vi "Best y for any element.vi"(7 "Enemys(T)\nAllys(F)":bool=TRUE, 9 "Maior intervalo(T)\nMaior angulo(F)":bool, 10 "IA State":T2={"our_robots"=[], "enemy_robots"=[], "balls"=[], "geometry"={"line_width"=0, "field_length"=0, "field_width"=0, "boundary_width"=0, "referee_width"=0, "goal_width"=0, "goal_depth"=0, "goal_wall_width"=0, "center_circle_radius"=0, "defense_radius"=0, "defense_stretch"=0, "free_kick_from_defense_dist"=0, "penalty_spot_from_field_line_dist"=0, "penalty_line_from_spot_dist"=0}, "IA Judge"={"stage"="", "command"="", "our_goalie_id"=0.0, "enemy_goalie_id"=0.0, "command enum"=enum."Halt", "Time"=enum."Azul"}, "Received Timestamp"=timestamp(0 s since 1904-01-01), "Events"={"Touch"=FALSE, "Ball out"=FALSE, "id touch"=0.0, "Ball out of \nVision"=FALSE, "Ball inside \nGoalie area"=FALSE, "Robot not responding"=FALSE, "Robots responding status"=[1.0, 1.0, 1.0, 1.0, 1.0, 1.0], "Enemy Ball \nPossession"=FALSE, "Pass State"=FALSE, "id end of pass"=0.0, "Kick"=FALSE, "Id ini Possession"=0.0, "Ball Possesion"=FALSE, "Id Possesion"=0.0, "Direct Kick"=FALSE, "2nd Strk Ativo"=FALSE}}, 11 "Element Position":dbl[](array[numeric])) -> (1 "Goal Gap Normalizado(%do gol aberta)":dbl, 2 "Best y(for kick target)":dbl, 3 "Goal Gap":dbl, 4 "Eclipse":bool, 5 "Gap Coord":dbl[](array[numeric]))   [LabVIEW 2017]
uses:
  Core/AI Input.ctl
  Core/AI Robot.ctl
  Intel/Functions Enum.ctl
  Intel/AttackerStates.ctl
  Path Planning/RRT/PathDests.ctl
  Path Planning/RRT/PathDest.ctl
  Core/AI Ball.ctl
  Core/Field Size.ctl
  Core/AI Judge.ctl
  Intel/Command Enum.ctl
  Events/Events.ctl
  segment.ctl
  <vilib>/Analysis/baseanly.llb/Real Dot Product.vi
  <vilib>/Analysis/NI_AALBase.lvlib
panel:
  out "Vetor de gaps \ncorreto":T1[](array[typedef])
  out "Vetor de gaps":T1[](array[typedef])
  in  "eclipse angle eps":dbl=0.035 format="%#_13g"
  out "pilha output (merged)":T1[](array[typedef])
  out "Vetor de segmentos ordenado":T1[](array[typedef])
  out "Vetor de segmentos (sombras)":T1[](array[typedef])
  # "Default FALSE"
  # "Quem será considerado obstaculo"
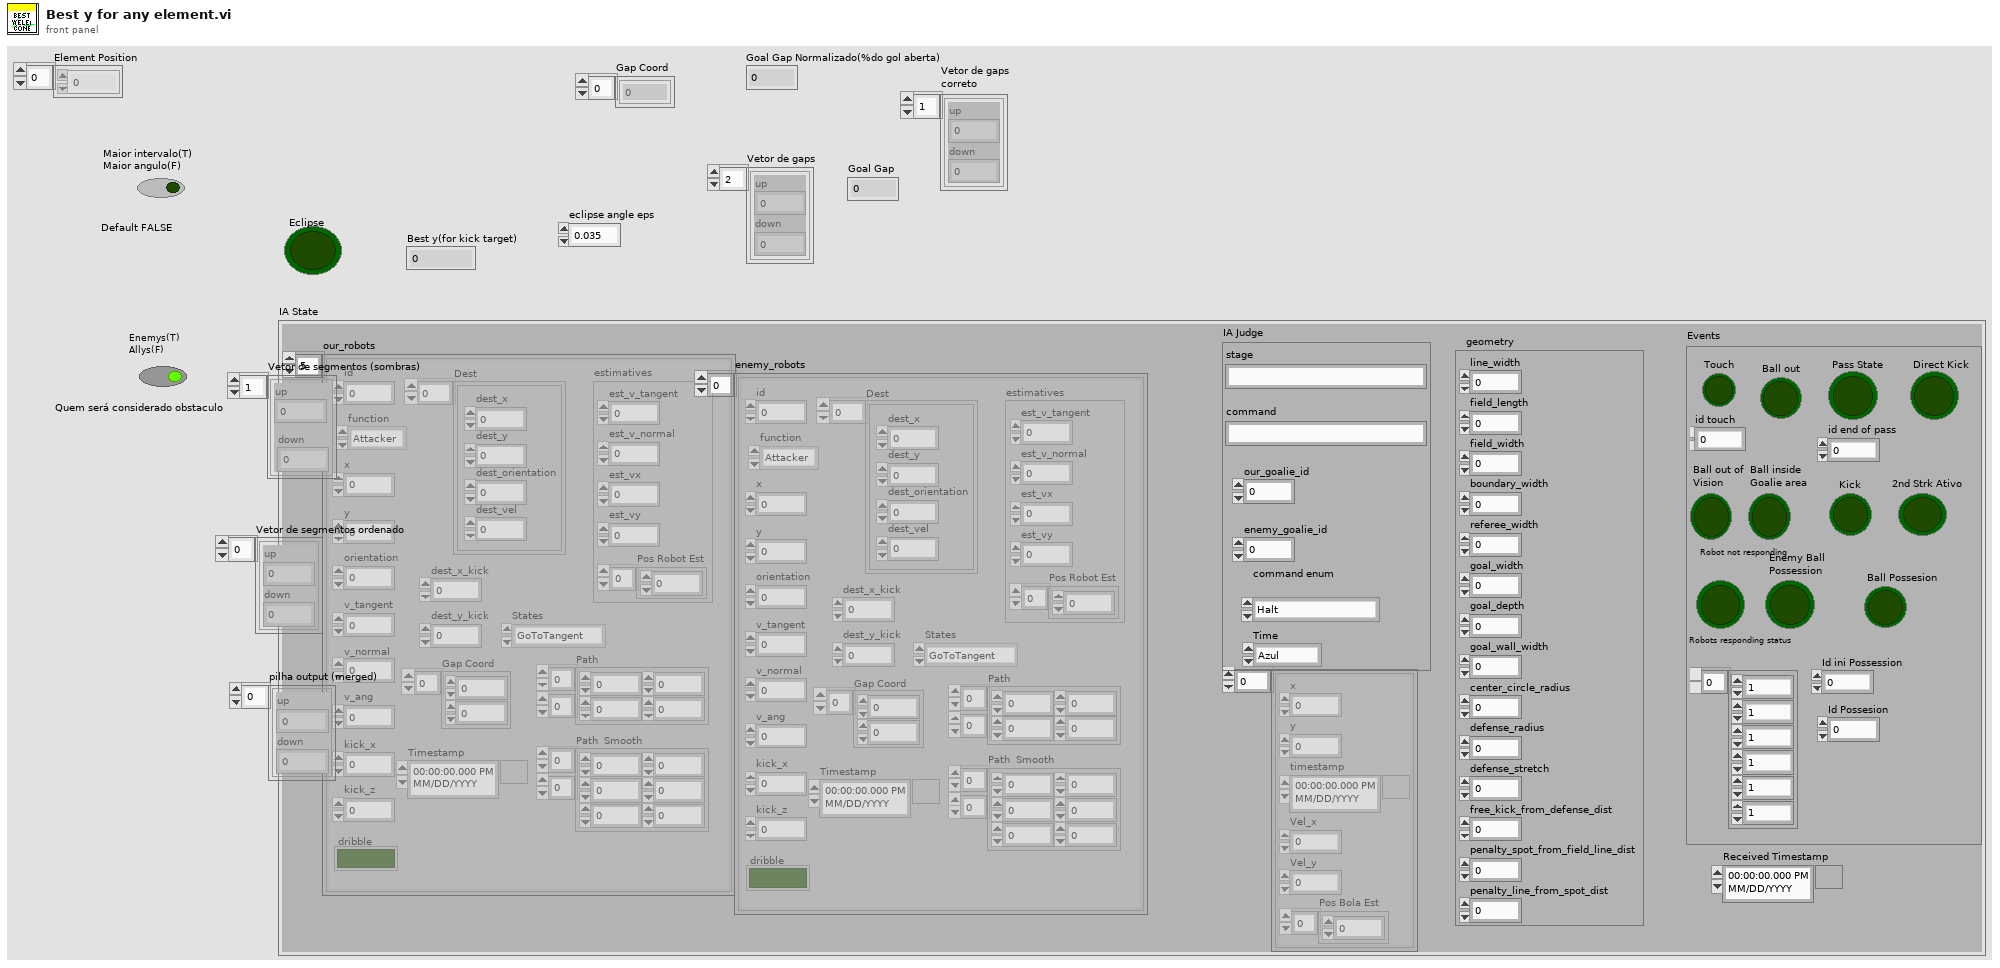
[diagram p1: front panel]
types:
  T1 = typedef "segment.ctl" = cluster{"up":dbl, "down":dbl}
  T2 = typedef "AI Input.ctl" = cluster{"our_robots":T3[], "enemy_robots":T3[], "balls":T8[], "geometry":T9, "IA Judge":T10, "Received Timestamp":timestamp, "Events":T12}
  T3 = typedef "AI Robot.ctl" = cluster{"id":u32, "function":T4, "x":dbl, "y":dbl, "orientation":dbl, "v_tangent":dbl, "v_normal":dbl, "v_ang":dbl, "kick_x":dbl, "kick_z":dbl, "dribble":bool, "Timestamp":timestamp, "estimatives":cluster{"est_v_tangent":dbl, "est_v_normal":dbl, "est_vx":dbl, "est_vy":dbl, "Pos Robot Est":dbl[]}, "dest_x_kick":dbl, "dest_y_kick":dbl, "Gap Coord":dbl[], "States":T5, "Path ":dbl[][], "Path  Smooth":dbl[][], "Dest":T6}
  T4 = typedef "Functions Enum.ctl" = enum16{"2nd Striker", "Attacker", "Goalie", "Defender", "Striker", "Goto 0", "Dummy", "Kicker", "ZigZag 0", "ZigZag 1", "ZigZag 2", "ZigZag 3", "ZigZag 4", "ZigZag 5", "ZigZag 6", "ZigZag 7", "ZigZag 8", ""}
  T5 = typedef "AttackerStates.ctl" = enum16{"Pass", "GoToTangent", "BallGetting", "GoToKick", ""}
  T6 = typedef "PathDests.ctl" = T7[]
  T7 = typedef "PathDest.ctl" = cluster{"dest_x":dbl, "dest_y":dbl, "dest_orientation":dbl, "dest_vel":dbl}
  T8 = typedef "AI Ball.ctl" = cluster{"x":dbl, "y":dbl, "timestamp":timestamp, "Vel_x":dbl, "Vel_y":dbl, "Pos Bola Est":dbl[]}
  T9 = typedef "Field Size.ctl" = cluster{"line_width":u32, "field_length":u32, "field_width":u32, "boundary_width":u32, "referee_width":u32, "goal_width":u32, "goal_depth":u32, "goal_wall_width":u32, "center_circle_radius":u32, "defense_radius":u32, "defense_stretch":u32, "free_kick_from_defense_dist":u32, "penalty_spot_from_field_line_dist":u32, "penalty_line_from_spot_dist":u32}
  T10 = typedef "AI Judge.ctl" = cluster{"stage":string, "command":string, "our_goalie_id":dbl, "enemy_goalie_id":dbl, "command enum":T11, "Time":enum16{"Azul", "Amarelo"}}
  T11 = typedef "Command Enum.ctl" = enum16{"Halt", "Stop", "Force Start", "PKA Normal Start", "Prepare Kickoff Ally", "PKE Normal Start", "Prepare Kickoff Enemy", "Prepare Penalty Ally", "PPA Normal Start", "Prepare Penalty Enemy", "PPE Normal Start", "Direct Free Enemy", "Direct Free Ally", "Indirect Free Enemy", "Indirect Free Ally", "Timeout Enemy", "Timeout Ally", "Goal Enemy", "Goal Ally", "Ball Placement Enemy", "Ball Placement Ally", "Normal Half Time", "Extra Time Break", "Extra Half Time", "None", "Post Game"}
  T12 = typedef "Events.ctl" = cluster{"Touch":bool, "Ball out":bool, "id touch":dbl, "Ball out of \nVision":bool, "Ball inside \nGoalie area":bool, "Robot not responding":bool, "Robots responding status":dbl[], "Enemy Ball \nPossession":bool, "Pass State":bool, "id end of pass":dbl, "Kick":bool, "Id ini Possession":dbl, "Ball Possesion":bool, "Id Possesion":dbl, "Direct Kick":bool, "2nd Strk Ativo":bool}
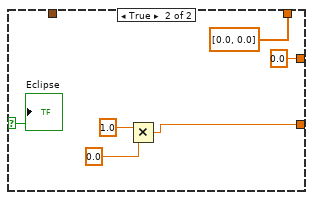
[diagram p4: hidden frame]
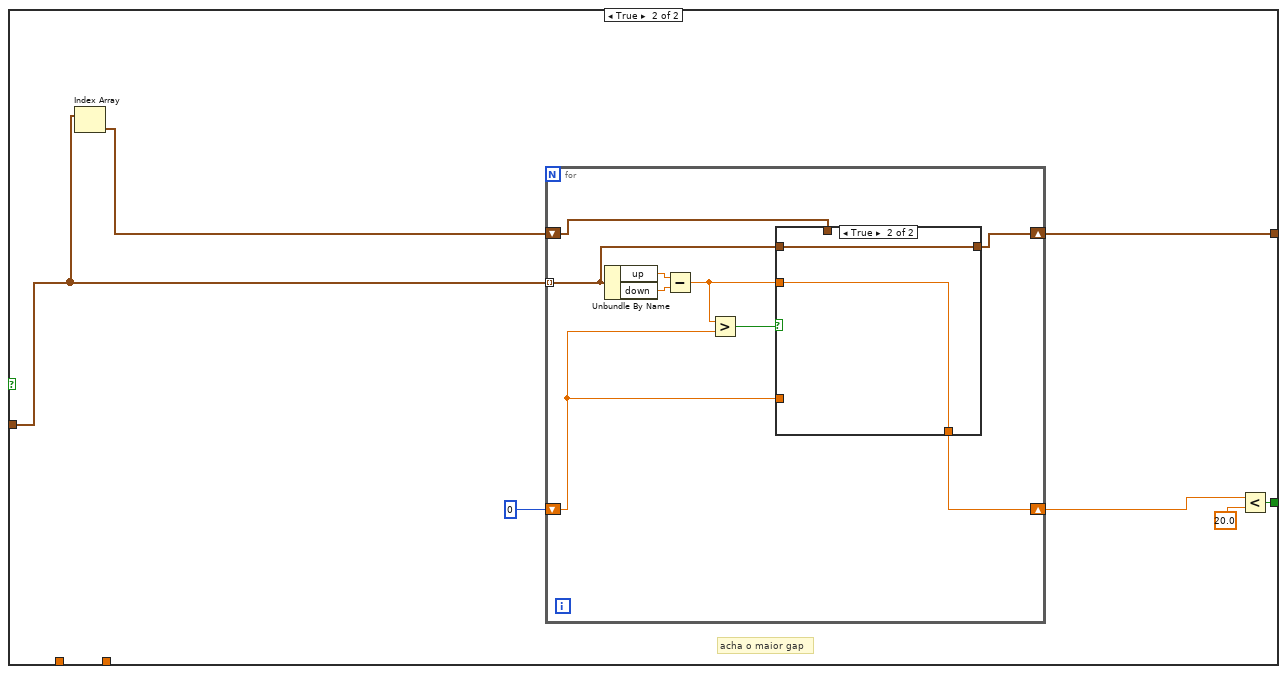
[diagram p6: hidden frame]
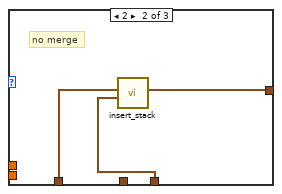
[diagram p8: hidden frame]
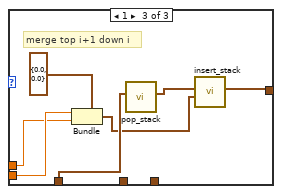
[diagram p9: hidden frame]
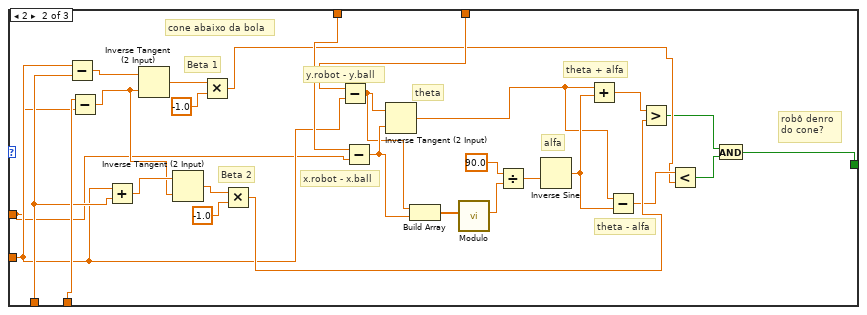
[diagram p11: hidden frame]
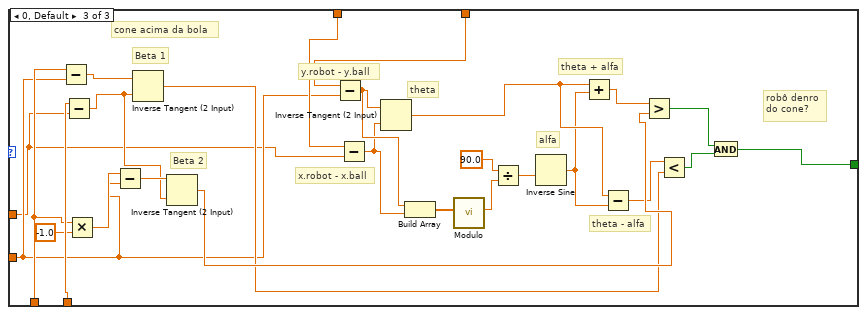
[diagram p12: hidden frame]
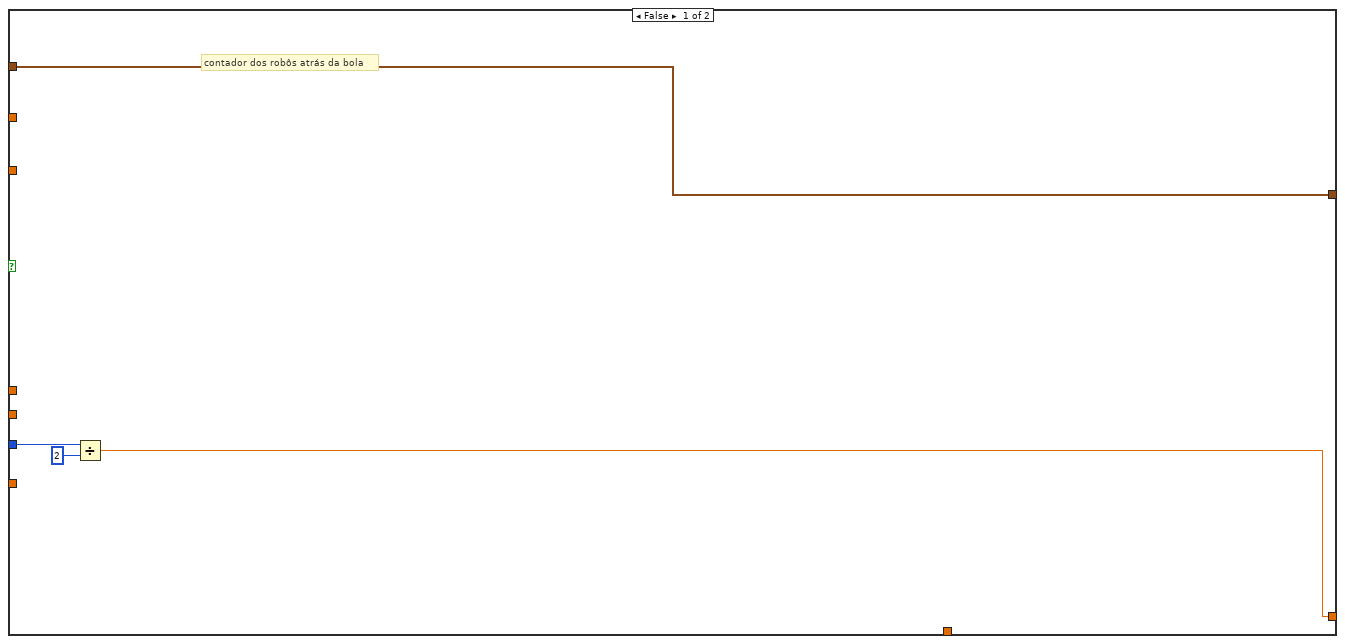
[diagram p13: hidden frame]
diagram:
  # "default T"
  # "Default FALSE"
  # "goal_width/2"
  # "field_length/2"
  # "balls"
  # "vetor de gaps"
  # "upper"
  n1 = Unbundle By Name("IA State") -> ("enemy_robots"=w21:T3[], "our_robots"=w20:T3[])
  n2 = Unbundle By Name("IA State") -> ("geometry.field_length"=w39:u32, "geometry.goal_width"=w2:u32)
  n3 = Select(t=w21, s="Enemys(T)\nAllys(F)", f=w20) -> (s? t:f=w19:T3[])
  n4 = Divide(x=w2, y=u32 2 ("x")) -> (x/y=w10:dbl)
  n5 = To Double Precision Float(number=w2) -> (double precision float=w1:dbl)
  n6 = for {
    shift-right: [w74] -> w24
    shift-left: T1[] [] -> [w73]
    tunnel: w39 -> [w51]
    tunnel: w10 -> [w53]
    tunnel: w10 -> [w71]
    shift-right: [w70] -> w22
    shift-left: _ -> [_]
    tunnel: w19 -> [w69] mode=indexing
    tunnel: "Enemys(T)\nAllys(F)" -> [w67]
    tunnel: "Element Position" -> [w43]
    # "y element"
    # "x element"
    # "y.robot"
    # "x.robot"
    # "field_length/2"
    # "goal_width/2"
    # "y element"
    # "x element"
    n7 = Index Array(array=w43) -> (element #1=w42:dbl, element #2=w41:dbl)  [unwired: 2 in]
    n8 = Unbundle By Name(w69) -> ("x"=w49:dbl, "y"=w48:dbl)
    n9 = Multiply(x=w49, y=-1.0) -> (x*y=w66:dbl)
    n10 = Absolute Value(x=w42) -> (abs(x)=w65:dbl)
    n11 = Absolute Value(x=w49) -> (abs(x)=w72:dbl)
    n12 = Select(t=w49, s=w67, f=w66) -> (s? t:f=w46:dbl)
    n13 = Greater?(x=w72, y=w65) -> (0:w44:bool)
    n14 = Multiply(x=w53, y=-1.0) -> (x*y=w57:dbl)
    n15 = Greater?(x=w41, y=w53) -> (0:w56:bool)
    n16 = Less?(x=w41, y=w57) -> (x < y?=w55:bool)
    n17 = Select(t=1, s=w56, f=0) -> (s? t:f=w63:i32)
    n18 = Select(t=0, s=w55, f=1) -> (s? t:f=w64:i32)
    n19 = Add(x=w63, y=w64) -> (x+y=w54:i32)
    n20 = Divide(x=w51, y=2.0) -> (x/y=w50:dbl)
    n21 = case shown="1" w54 {
      tunnel: w53 -> [w77 w103 w151]
      tunnel: w50 -> [w98 w123 w153]
      tunnel: w46 -> [w85 w110 w146]
      tunnel: w48 -> [w84 w111 w147]
      tunnel: [w86 w112 w137] -> w45
      tunnel: w42 -> [w75 w101 w129]
      tunnel: w41 -> [w76 w102 w130]
      frame 1 {
        # "robô denro\ndo cone?"
        # "cone centrado"
        # "theta - alfa"
        # "theta + alfa"
        # "theta"
        # "alfa"
        # "x.robot - x.element"
        # "y.robot - y.element"
        # "Beta 2"
        # "Beta 1"
        n22 = Subtract(x=w77, y=w76) -> (x-y=w99:dbl)
        n23 = Subtract(x=w98, y=w75) -> (x-y=w100:dbl)
        n24 = Add(x=w76, y=w77) -> (x+y=w97:dbl)
        n25 = Inverse Tangent (2 Input)(1:w100, 2:w99) -> (0:w80:dbl)
        n26 = Inverse Tangent (2 Input)(1:w100, 2:w97) -> (0:w96:dbl)
        n27 = Multiply(x=w96, y=-1.0) -> (x*y=w82:dbl)
        n28 = Subtract(x=w84, y=w76) -> (x-y=w87:dbl)
        n29 = Subtract(x=w85, y=w75) -> (x-y=w88:dbl)
        n30 = Inverse Tangent (2 Input)(1:w88, 2:w87) -> (0:w93:dbl)
        n31 = Build Array(w87, w88) -> (w89:dbl[])
        n32 = call "Modulo.vi"("2D vector"=w89) -> ("Modulo"=w90:dbl)  [unwired: 10 in]
        n33 = Divide(x=90.0, y=w90) -> (x/y=w91:dbl)
        n34 = Inverse Sine(1:w91) -> (0:w94:dbl)
        n35 = Add(x=w93, y=w94) -> (x+y=w83:dbl)
        n36 = Subtract(x=w93, y=w94) -> (x-y=w81:dbl)
        n37 = Greater?(x=w83, y=w82) -> (0:w78:bool)
        n38 = Less?(x=w81, y=w80) -> (x < y?=w79:bool)
        n39 = And(x=w78, y=w79) -> (x .and. y?=w86:bool)
      }
      frame 2 {
        # "robô denro\ndo cone?"
        # "cone abaixo da bola"
        # "theta - alfa"
        # "theta + alfa"
        # "theta"
        # "alfa"
        # "x.robot - x.ball"
        # "y.robot - y.ball"
        # "Beta 2"
        # "Beta 1"
        n40 = Subtract(x=w102, y=w103) -> (x-y=w125:dbl)
        n41 = Subtract(x=w123, y=w101) -> (x-y=w124:dbl)
        n42 = Add(x=w102, y=w103) -> (x+y=w126:dbl)
        n43 = Inverse Tangent (2 Input)(1:w124, 2:w125) -> (0:w121:dbl)
        n44 = Inverse Tangent (2 Input)(1:w124, 2:w126) -> (0:w127:dbl)
        n45 = Multiply(x=w121, y=-1.0) -> (x*y=w106:dbl)
        n46 = Multiply(x=w127, y=-1.0) -> (x*y=w108:dbl)
        n47 = Subtract(x=w111, y=w102) -> (x-y=w113:dbl)
        n48 = Subtract(x=w110, y=w101) -> (x-y=w114:dbl)
        n49 = Inverse Tangent (2 Input)(1:w114, 2:w113) -> (0:w119:dbl)
        n50 = Build Array(w113, w114) -> (w115:dbl[])
        n51 = call "Modulo.vi"("2D vector"=w115) -> ("Modulo"=w116:dbl)  [unwired: 10 in]
        n52 = Divide(x=90.0, y=w116) -> (x/y=w117:dbl)
        n53 = Inverse Sine(1:w117) -> (0:w120:dbl)
        n54 = Add(x=w119, y=w120) -> (x+y=w109:dbl)
        n55 = Subtract(x=w119, y=w120) -> (x-y=w107:dbl)
        n56 = Greater?(x=w109, y=w108) -> (0:w104:bool)
        n57 = Less?(x=w107, y=w106) -> (x < y?=w105:bool)
        n58 = And(x=w104, y=w105) -> (x .and. y?=w112:bool)
      }
      frame 0, Default {
        # "robô denro\ndo cone?"
        # "cone acima da bola"
        # "theta - alfa"
        # "theta + alfa"
        # "theta"
        # "alfa"
        # "x.robot - x.ball"
        # "y.robot - y.ball"
        # "Beta 2"
        # "Beta 1"
        n59 = Subtract(x=w151, y=w130) -> (x-y=w154:dbl)
        n60 = Subtract(x=w153, y=w129) -> (x-y=w148:dbl)
        n61 = Multiply(x=w151, y=-1.0) -> (x*y=w150:dbl)
        n62 = Subtract(x=w150, y=w130) -> (x-y=w149:dbl)
        n63 = Inverse Tangent (2 Input)(1:w148, 2:w154) -> (0:w132:dbl)
        n64 = Inverse Tangent (2 Input)(1:w148, 2:w149) -> (0:w135:dbl)
        n65 = Subtract(x=w147, y=w130) -> (x-y=w145:dbl)
        n66 = Subtract(x=w146, y=w129) -> (x-y=w144:dbl)
        n67 = Inverse Tangent (2 Input)(1:w144, 2:w145) -> (0:w139:dbl)
        n68 = Build Array(w145, w144) -> (w143:dbl[])
        n69 = call "Modulo.vi"("2D vector"=w143) -> ("Modulo"=w142:dbl)  [unwired: 10 in]
        n70 = Divide(x=90.0, y=w142) -> (x/y=w141:dbl)
        n71 = Inverse Sine(1:w141) -> (0:w138:dbl)
        n72 = Add(x=w139, y=w138) -> (x+y=w136:dbl)
        n73 = Subtract(x=w139, y=w138) -> (x-y=w133:dbl)
        n74 = Greater?(x=w136, y=w135) -> (0:w134:bool)
        n75 = Less?(x=w133, y=w132) -> (x < y?=w131:bool)
        n76 = And(x=w134, y=w131) -> (x .and. y?=w137:bool)
      }
    }
    n77 = And(x=w44, y=w45) -> (x .and. y?=w47:bool)
    n78 = case shown="True" w47 {
      tunnel: [w158 w165] -> w74
      tunnel: w73 -> [w158 w167]
      tunnel: w51 -> [w157 w172]
      tunnel: w53 -> [_ w171]
      tunnel: w71 -> [_ w164]
      tunnel: [w155 w163] -> w70
      tunnel: w48 -> [_ w162]
      tunnel: w46 -> [_ w161]
      tunnel: w42 -> [_ w159]
      tunnel: w41 -> [_ w160]
      frame False {
        # "contador dos robôs atrás da bola"
        n79 = Divide(x=w157, y=u32 2) -> (x/y=w155:dbl)
      }
      frame True {
        n80 = flat-sequence {
          tunnel: w162 -> [w207]
          tunnel: w172 -> [w203]
          tunnel: w171 -> [w188]
          tunnel: [w178] -> w170
          tunnel: [w177] -> w169
          tunnel: [w189] -> w168
          tunnel: w167 -> [w182]
          tunnel: [w182] -> w166
          tunnel: [w176] -> w163
          tunnel: w161 -> [w175]
          tunnel: w160 -> [w173]
          tunnel: w159 -> [w174]
          tunnel: w170 -> [w211]
          tunnel: w169 -> [w210]
          tunnel: w168 -> [w212]
          tunnel: w166 -> [w213]
          tunnel: [w209] -> w165
          tunnel: w164 -> [w208]
          frame #0 {
            # "theta - alfa"
            # "alfa + theta"
            # "theta"
            # "alfa"
            # "x.robot - x.element"
            # "y.robot - y.element"
            n81 = Divide(x=w203, y=u32 2 ("x")) -> (x/y=w176:dbl)
            n82 = Subtract(x=w175, y=w174) -> (x-y=w186:dbl)
            n83 = Subtract(x=w207, y=w173) -> (x-y=w187:dbl)
            n84 = Multiply(x=w188, y=-1.0) -> (x*y=w194:dbl)
            n85 = Subtract(x=w176, y=w174) -> (x-y=w179:dbl)
            n86 = Inverse Tangent (2 Input)(1:w186, 2:w187) -> (0:w185:dbl)
            n87 = Build Array(w187, w186) -> (w206:dbl[])
            n88 = call "Modulo.vi"("2D vector"=w206) -> ("Modulo"=w204:dbl)  [unwired: 10 in]
            n89 = Divide(x=90.0, y=w204) -> (x/y=w184:dbl)
            n90 = Inverse Sine(1:w184) -> (0:w183:dbl)
            n91 = Subtract(x=w185, y=w183) -> (x-y=w199:dbl)
            n92 = Tangent(1:w199) -> (0:w198:dbl)
            n93 = Add(x=w185, y=w183) -> (x+y=w201:dbl)
            n94 = Tangent(1:w201) -> (0:w200:dbl)
            n95 = Multiply(x=w198, y=w179) -> (x*y=w180:dbl)
            n96 = Multiply(x=w200, y=w179) -> (x*y=w181:dbl)
            n97 = Add(x=w180, y=w173) -> (x+y=w177:dbl)
            n98 = Add(x=w181, y=w173) -> (x+y=w178:dbl)
            n99 = Less?(x=w178, y=w194) -> (x < y?=w193:bool)
            n100 = Less?(x=w177, y=w194) -> (x < y?=w192:bool)
            n101 = Greater?(x=w177, y=w188) -> (0:w196:bool)
            n102 = Greater?(x=w178, y=w188) -> (0:w197:bool)
            n103 = And(x=w197, y=w196) -> (x .and. y?=w191:bool)
            n104 = And(x=w193, y=w192) -> (x .and. y?=w190:bool)
            n105 = Or(x=w191, y=w190) -> (x .or. y?=w189:bool)
          }
          frame #1 {
            # "goal_width/2"
            n106 = case shown="False" w212 {
              tunnel: [w222 w225] -> w209
              tunnel: w213 -> [w221 w225]
              tunnel: w211 -> [w220 _]
              tunnel: w210 -> [w218 _]
              tunnel: w208 -> [w217 _]
              frame False {
                n107 = Max & Min(x=w220, y=w217) -> (min(x,y)=w219:dbl)  [unwired: 1 out]
                n108 = Multiply(x=w217, y=-1.0) -> (x*y=w215:dbl)
                n109 = Max & Min(x=w218, y=w215) -> (max(x,y)=w214:dbl)  [unwired: 1 out]
                n110 = Bundle(cluster=T1 {"up"=0.0, "down"=0.0} ("segment 2"), "up"=w219, "down"=w214) -> (w223:T1)
                n111 = Insert Into Array(array=w221, new element=w223) -> (w222:T1[])  [unwired: 1 in]
              }
              frame True {
              }
            }
          }
        }
      }
    }
  }
  "Vetor de segmentos (sombras)" <- w24
  n112 = Sort 1D Array(array=w24) -> (sorted array=w36:T1[])
  "Vetor de segmentos ordenado" <- w36
  n113 = Index Array(array=w36) -> (element=w35:T1)  [unwired: 1 in]
  n114 = call "insert_stack.vi"("novo elemento"=w35, "pilha input"=T1[] []) -> ("pilha output"=w33:T1[])  [unwired: 9 in]
  n115 = for {
    shift-right: [w226] -> w32
    shift-left: w33 -> [w228]
    tunnel: w36 -> [w227] mode=indexing
    i -> [w229]
    n116 = case shown="Default" w229 {
      tunnel: w228 -> [w233 w261]
      tunnel: w227 -> [w236 _]
      tunnel: [w234 w261] -> w226
      frame Default {
        # "pilha"
        # "i+1"
        # "i"
        # "i+1"
        # "i"
        n117 = call "top_stack.vi"("pilha input"=w233) -> ("top"=w235:T1)  [unwired: 10 in]
        n118 = Unbundle By Name(w235) -> ("up"=w232:dbl, "down"=w237:dbl)
        n119 = Unbundle By Name(w236) -> ("down"=w231:dbl, "up"=w238:dbl)
        n120 = Greater Or Equal?(x=w231, y=w232) -> (x >= y?=w230:bool)
        n121 = Less?(x=w231, y=w237) -> (x < y?=w240:bool)
        n122 = Select(t=1, s=w230, f=0) -> (s? t:f=w242:i32)
        n123 = Select(t=0, s=w240, f=1) -> (s? t:f=w241:i32)
        n124 = Add(x=w242, y=w241) -> (x+y=w239:i32)
        n125 = case shown="0, Default" w239 {
          tunnel: w238 -> [_ _ w259]
          tunnel: w237 -> [_ _ w258]
          tunnel: w235 -> [_ _ _]
          tunnel: w236 -> [w247 w252 _]
          tunnel: [w250 w251 w254] -> w234
          tunnel: w233 -> [w249 w253 w257]
          frame 0, Default {
            # "merge:  i+1"
            n126 = call "pop_stack.vi"("pilha input"=w249) -> ("pilha output"=w248:T1[])  [unwired: 9 in]
            n127 = call "insert_stack.vi"("novo elemento"=w247, "pilha input"=w248) -> ("pilha output"=w250:T1[])  [unwired: 9 in]
          }
          frame 2 {
            # "no merge"
            n128 = call "insert_stack.vi"("novo elemento"=w252, "pilha input"=w253) -> ("pilha output"=w251:T1[])  [unwired: 9 in]
          }
          frame 1 {
            # "merge top i+1 down i"
            n129 = Bundle(cluster=T1 {"up"=0.0, "down"=0.0} ("segment 2"), "up"=w259, "down"=w258) -> (w255:T1)
            n130 = call "pop_stack.vi"("pilha input"=w257) -> ("pilha output"=w256:T1[])  [unwired: 9 in]
            n131 = call "insert_stack.vi"("novo elemento"=w255, "pilha input"=w256) -> ("pilha output"=w254:T1[])  [unwired: 9 in]
          }
        }
      }
      frame 0 {
      }
    }
  }
  "pilha output (merged)" <- w32
  n132 = Reverse 1D Array(array=w32) -> (reversed array=w31:T1[])
  n133 = for {
    tunnel: w31 -> [w269] mode=indexing
    shift-right: [w263] -> w28
    shift-left: T1[] [] -> [w265]
    shift-right: [w264] -> w27
    shift-left: w10 -> [w266]
    n134 = Unbundle By Name(w269) -> ("up"=w262:dbl, "down"=w264:dbl)
    n135 = Bundle(cluster=T1 {"up"=0.0, "down"=0.0} ("segment 2"), "up"=w266, "down"=w262) -> (w268:T1)
    n136 = Insert Into Array(array=w265, new element=w268) -> (w263:T1[])  [unwired: 1 in]
  }
  n137 = Multiply(x=w10, y=-1.0) -> (x*y=w25:dbl)
  n138 = Bundle(cluster=T1 {"up"=0.0, "down"=0.0} ("segment 2"), "up"=w27, "down"=w25) -> (w30:T1)
  n139 = Insert Into Array(array=w28, new element=w30) -> (w11:T1[])  [unwired: 1 in]
  n140 = Array Size(array=w11) -> (size(s)=w13:i32)
  n141 = Decrement(x=w13) -> (x-1=w12:i32)
  n142 = for {
    N: w12 -> [_]
    shift-right: [w270] -> w9
    shift-left: w11 -> [w272]
    i -> [w271]
    n143 = Increment(x=w271) -> (x+1=w280:i32)
    n144 = Index Array(array=w272, index=w271) -> (element=w273:T1)
    n145 = Index Array(array=w272, index=w280) -> (element=w279:T1)
    n146 = Unbundle By Name(w279) -> ("up"=w277:dbl, "down"=w274:dbl)
    n147 = Unbundle By Name(w273) -> ("up"=w275:dbl, "down"=w278:dbl)
    n148 = Equal?(x=w278, y=w277) -> (x = y?=w276:bool)
    n149 = case shown="True" w276 {
      tunnel: w275 -> [_ w290]
      tunnel: w274 -> [_ w289]
      tunnel: w273 -> [_ w288]
      tunnel: w272 -> [w281 w286]
      tunnel: w271 -> [_ w283]
      tunnel: [w281 w282] -> w270
      frame False {
      }
      frame True {
        n150 = Bundle By Name(cluster=w288, "up"=w290, "down"=w289) -> (w284:T1)
        n151 = Delete From Array(array=w286, length=2, index=w283) -> (array with subset deleted=w285:T1[])  [unwired: 1 out]
        n152 = Insert Into Array(array=w285, index=w283, new element=w284) -> (w282:T1[])
      }
    }
  }
  "Vetor de gaps" <- w9
  n153 = for {
    tunnel: w10 -> [w300]
    tunnel: w9 -> [w293] mode=indexing
    shift-right: [w295] -> w6
    shift-left: T1[] [] -> [w294]
    n154 = Unbundle By Name(w293) -> ("up"=w292:dbl, "down"=w291:dbl)
    n155 = Multiply(x=w300, y=-1.0) -> (x*y=w299:dbl)
    n156 = Greater?(x=w292, y=w300) -> (0:w297:bool)
    n157 = Less?(x=w291, y=w299) -> (x < y?=w296:bool)
    n158 = Or(x=w297, y=w296) -> (x .or. y?=w298:bool)
    n159 = case shown="False" w298 {
      tunnel: [w302 w305] -> w295
      tunnel: w294 -> [w302 w306]
      tunnel: w292 -> [_ w303]
      tunnel: w291 -> [_ w304]
      frame True {
      }
      frame False {
        n160 = Bundle(cluster=T1 {"up"=0.0, "down"=0.0} ("segment 2"), "up"=w303, "down"=w304) -> (w307:T1)
        n161 = Insert Into Array(array=w306, new element=w307) -> (w305:T1[])  [unwired: 1 in]
      }
    }
  }
  "Vetor de gaps \ncorreto" <- w6
  n162 = case shown="False" "Maior intervalo(T)\nMaior angulo(F)" {
    tunnel: [w313 w349] -> w16
    tunnel: [w312 w347] -> w17
    tunnel: w6 -> [w317 w348]
    tunnel: w22 -> [w316 _]
    tunnel: "Element Position" -> [w311 _]
    frame False {
      # "acha o maior ângulo"
      n163 = Index Array(array=w311) -> (element #1=w310:dbl, element #2=w309:dbl)  [unwired: 2 in]
      n164 = Index Array(array=w317) -> (element=w318:T1)  [unwired: 1 in]
      n165 = for {
        tunnel: w317 -> [w339] mode=indexing
        shift-right: [w340] -> w315
        shift-left: 0 -> [w322]
        shift-right: [w338] -> w312
        shift-left: w318 -> [w337]
        tunnel: w310 -> [w321]
        tunnel: w309 -> [w320]
        tunnel: w316 -> [w336]
        # "theta"
        # "cos (theta)"
        # "vetor bola-down"
        # "vetor bola-up"
        n166 = Unbundle By Name(w339) -> ("up"=w335:dbl, "down"=w332:dbl)
        n167 = Subtract(x=w336, y=w321) -> (x-y=w333:dbl)
        n168 = Subtract(x=w332, y=w320) -> (x-y=w331:dbl)
        n169 = Subtract(x=w335, y=w320) -> (x-y=w334:dbl)
        n170 = Build Array(w333, w331) -> (w329:dbl[])
        n171 = Build Array(w333, w334) -> (w330:dbl[])
        n172 = call-poly <vilib>:"Dot Product.vi"("Y Vector"=w329, "X Vector"=w330) -> ("X * Y"=w326:dbl)  [unwired: 1 out]
        n173 = call "Modulo.vi"("2D vector"=w330) -> ("Modulo"=w328:dbl)  [unwired: 10 in]
        n174 = call "Modulo.vi"("2D vector"=w329) -> ("Modulo"=w327:dbl)  [unwired: 10 in]
        n175 = Multiply(x=w328, y=w327) -> (x*y=w325:dbl)
        n176 = Divide(x=w326, y=w325) -> (x/y=w324:dbl)
        n177 = Inverse Cosine(1:w324) -> (0:w323:dbl)
        n178 = Greater?(x=w323, y=w322) -> (0:w341:bool)
        n179 = case shown="True" w341 {
          tunnel: w323 -> [_ w345]
          tunnel: [w342 w345] -> w340
          tunnel: w339 -> [_ w344]
          tunnel: [w343 w344] -> w338
          tunnel: w337 -> [w343 _]
          tunnel: w322 -> [w342 _]
          frame False {
          }
          frame True {
          }
        }
      }
      n180 = Less?(x=w315, y="eclipse angle eps") -> (x < y?=w313:bool)
    }
    frame True {
      # "acha o maior gap"
      n181 = Index Array(array=w348) -> (element=w351:T1)  [unwired: 1 in]
      n182 = for {
        tunnel: w348 -> [w356] mode=indexing
        shift-right: [w357] -> w350
        shift-left: 0 -> [w354]
        shift-right: [w355] -> w347
        shift-left: w351 -> [w353]
        n183 = Unbundle By Name(w356) -> ("up"=w361:dbl, "down"=w360:dbl)
        n184 = Subtract(x=w361, y=w360) -> (x-y=w358:dbl)
        n185 = Greater?(x=w358, y=w354) -> (0:w359:bool)
        n186 = case shown="True" w359 {
          tunnel: w358 -> [_ w365]
          tunnel: [w363 w365] -> w357
          tunnel: w356 -> [_ w364]
          tunnel: [w362 w364] -> w355
          tunnel: w354 -> [w363 _]
          tunnel: w353 -> [w362 _]
          frame False {
          }
          frame True {
          }
        }
      }
      n187 = Less?(x=w350, y=20.0) -> (x < y?=w349:bool)
    }
  }
  n188 = case shown="False" w16 {
    selector: w16 -> [_ w380]
    tunnel: w17 -> [w372 _]
    tunnel: [w371 w377] -> w14
    tunnel: [w369 0.0] -> w3
    tunnel: [w366 dbl[] [0.0, 0.0] ("Gap Coord")] -> w15
    frame False {
      n189 = Unbundle By Name(w372) -> ("up"=w368:dbl, "down"=w367:dbl)
      n190 = Subtract(x=w368, y=w367) -> (x-y=w370:dbl)
      n191 = Build Array(w368, w367) -> (w366:dbl[])
      n192 = Add(x=w368, y=w367) -> (x+y=w373:dbl)
      n193 = Absolute Value(x=w370) -> (abs(x)=w369:dbl)
      n194 = Divide(x=w373, y=2.0) -> (x/y=w371:dbl)
    }
    frame True {
      n195 = Multiply(x=1.0, y=0.0) -> (x*y=w377:dbl)
      "Eclipse" <- w380
    }
  }
  "Best y(for kick target)" <- w14
  "Goal Gap" <- w3
  "Gap Coord" <- w15
  n196 = Divide(x=w3, y=w1) -> (x/y=→"Goal Gap Normalizado(%do gol aberta)":dbl)
